vi "题目四.vi"() -> ()   [LabVIEW 2017]
panel:
  in  "停止":bool
  in  "枚举":enum16{"王五", "李四", "张三"}(ring)
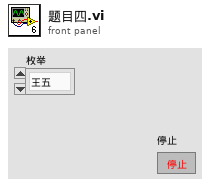
[diagram p1: front panel]
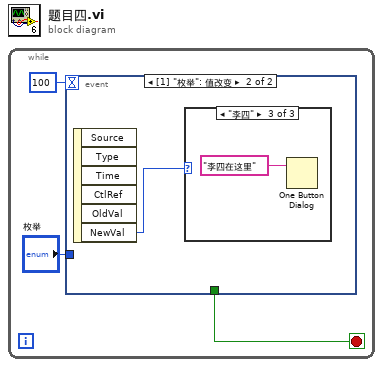
[diagram p0: block diagram]
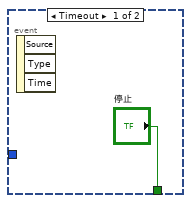
[diagram p2: hidden frame]
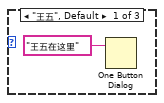
[diagram p3: hidden frame]
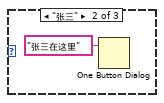
[diagram p4: hidden frame]
diagram:
  n1 = while {
    stop <- w2 stop-if-true
    n2 = event shown="[1] \"枚举\": 值改变" {
      selector: _ -> [_ _]
      dyn-events: _ -> [_ _]
      timeout: 100 -> [_ _]
      tunnel: ["停止" _] -> w2
      tunnel: "枚举" -> [_ _]
      event Timeout {
        n3 = event-data() -> ()  [unwired: 1 in, 3 out]
      }
      event "枚举": Value Change {
        n4 = event-data() -> ("NewVal"=w5:enum16{"王五", "李四", "张三"})  [unwired: 1 in, 5 out]
        n5 = case shown="\"李四\"" w5 {
          frame "王五", Default {
            n6 = One Button Dialog(message="王五在这里") -> ()  [unwired: 1 in, 1 out]
          }
          frame "张三" {
            n7 = One Button Dialog(message="张三在这里") -> ()  [unwired: 1 in, 1 out]
          }
          frame "李四" {
            n8 = One Button Dialog(message="李四在这里") -> ()  [unwired: 1 in, 1 out]
          }
        }
      }
    }
  }
